vi "2nd channel add delete.vi"(9 "action":enum16{"delete", "insert"}(ring), 10 "Index":u32, 11 "Calibration array":T1 {"D.O."."K" format="%.6f"; "D.O."."Temperature" format="%.2f"; "pH scale"."Buffers"."V/T" format="%.5f"; "pH scale"."Buffers"."Buffer" format="%.2f"; "pH scale"."Temperature" format="%.2f"; "offset (physical units)" format="%.5f"; "correspondence table"."volts" format="%.4f"; "correspondence table"."physical units" format="%.4f"; "second channel" min=-1; "offset (volts)" format="%.5f"; "conversion matrix" format="%.4e"}) -> (3 "Calibration array out":T1 {"D.O."."K" format="%.6f"; "D.O."."Temperature" format="%.2f"; "pH scale"."Buffers"."V/T" format="%.5f"; "pH scale"."Buffers"."Buffer" format="%.2f"; "pH scale"."Temperature" format="%.2f"; "offset (physical units)" format="%.5f"; "correspondence table"."volts" format="%.4f"; "correspondence table"."physical units" format="%.4f"; "second channel" min=-1; "offset (volts)" format="%.5f"; "conversion matrix" format="%.4e"})   [LabVIEW 2012]
uses:
  calib array.ctl
  conversion.ctl
  DAQ configuration/scale type.ctl
  correspondence table.ctl
  pH/pH scale.ctl
  Dissolved Oxygen/DO scale.ctl
panel:
  # "C"
  # "kPa"
  # "C"
  # "C"
  # "kPa"
  # "C"
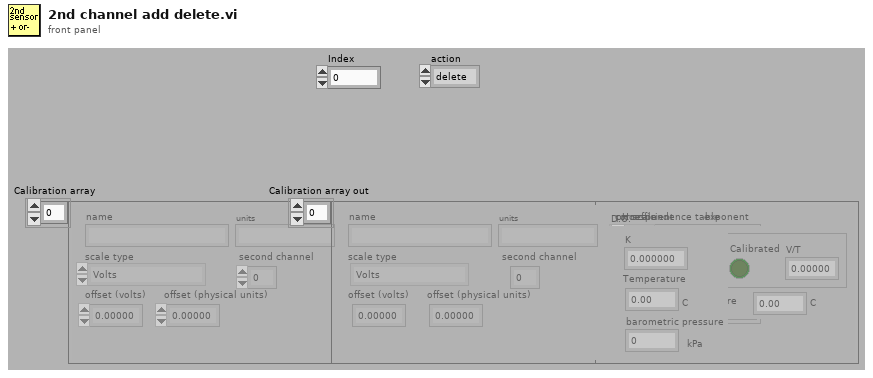
[diagram p1: front panel]
types:
  T1 = typedef "calib array.ctl" = T2[]
  T2 = typedef "conversion.ctl" = cluster{"conversion matrix":sgl[][], "units":string, "name":string, "scale type":T3, "offset (volts)":dbl, "second channel":i8, "correspondence table":T4, "offset (physical units)":dbl, "pH scale":T5, "D.O.":T6}
  T3 = typedef "scale type.ctl" = enum16{"Volts", "Polynomial", "Correspondence Table", "pH", "Dissolved Oxygen", "Quadratic"}
  T4 = typedef "correspondence table.ctl" = cluster{"physical units":dbl, "volts":dbl}[]
  T5 = typedef "pH scale.ctl" = cluster{"Buffers":cluster{"Buffer":dbl, "Calibrated":bool, "V/T":dbl}[], "Temperature":dbl}
  T6 = typedef "DO scale.ctl" = cluster{"Temperature":dbl, "K":dbl, "barometric pressure":dbl}
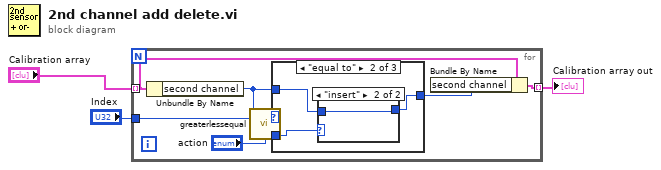
[diagram p0: block diagram]
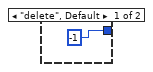
[diagram p3: hidden frame]
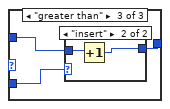
[diagram p4: hidden frame]
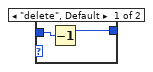
[diagram p5: hidden frame]
diagram:
  n1 = for {
    tunnel: "Calibration array" -> [w10] mode=indexing
    tunnel: "Index" -> [w8]
    tunnel: [w9] -> w1 mode=indexing
    n2 = Unbundle By Name(w10) -> ("second channel"=w5:i8)
    n3 = call "greaterlessequal.vi"("y"=w8, "x"=w5) -> ("comparison"=w7:enum16{"less than", "equal to", "greater than"})  [unwired: 9 in]
    n4 = case shown="\"equal to\"" w7 {
      tunnel: [w11 w13 w18] -> w6
      tunnel: w5 -> [w11 w12 w19]
      tunnel: "action" -> [_ w14 w17]
      frame "less than", Default {
      }
      frame "equal to" {
        n5 = case shown="\"insert\"" w14 {
          tunnel: w12 -> [_ w16]
          tunnel: [-1 w16] -> w13
          frame "delete", Default {
          }
          frame "insert" {
          }
        }
      }
      frame "greater than" {
        n6 = case shown="\"insert\"" w17 {
          tunnel: w19 -> [w21 w23]
          tunnel: [w20 w22] -> w18
          frame "delete", Default {
            n7 = Decrement(x=w21) -> (x-1=w20:i8)
          }
          frame "insert" {
            n8 = Increment(x=w23) -> (x+1=w22:i8)
          }
        }
      }
    }
    n9 = Bundle By Name(cluster=w10, "second channel"=w6) -> (w9:T2)
  }
  "Calibration array out" <- w1
